vi "LNLS Control PS Data to LOCON_BIPOLAR_16BITS Data_Command9.vi"(8 "error in (no error)":errorcluster, 9 "PS Status (On correction?)":bool[](array[boolean]), 10 "PS Status (ON/OFF)":bool[](array[boolean]), 11 "PS Readings/Setpoints":dbl[](array[numeric])) -> (0 "error out":errorcluster, 3 "PS Readings/Setpoints LOCON Data":T1[](array[typedef]) {"status" format="%08b"})   [LabVIEW 2011, in "LNLS Control VIs.lvlib"]
uses:
  Types Definitions/Type LOCON_BIPOLAR_16BITS.ctl
  LNLS Control VIs.lvlib
  Type Definitions.lvlib
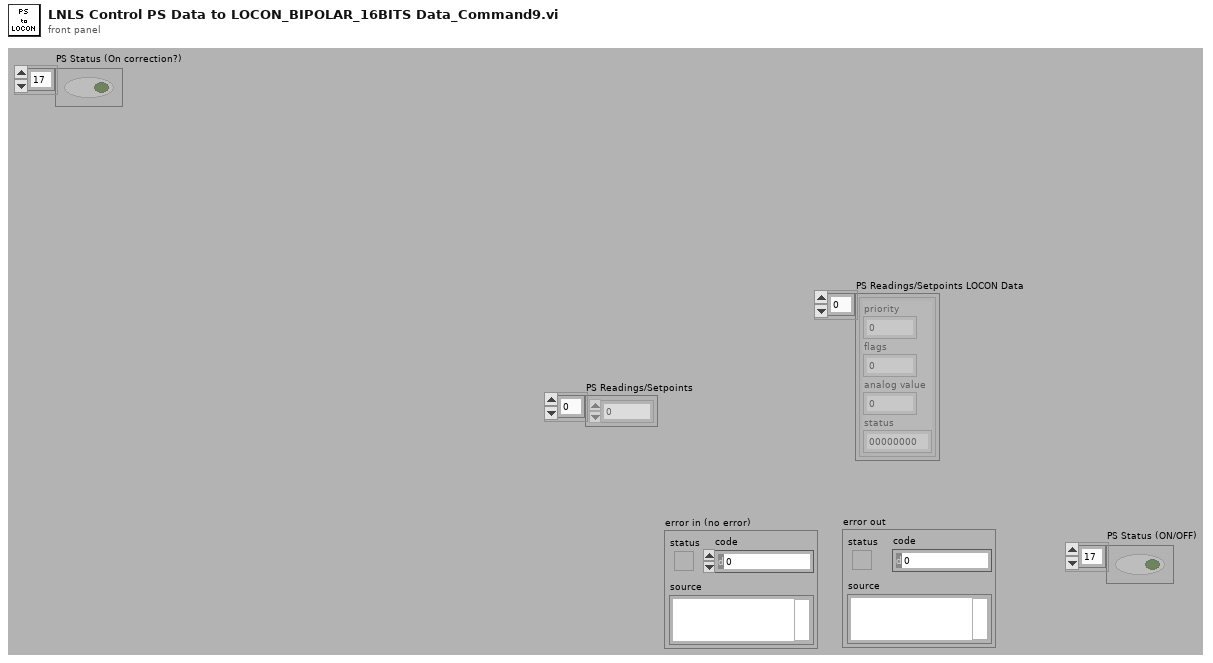
[diagram p1: front panel]
types:
  T1 = typedef "Type Definitions.lvlib/Type LOCON_BIPOLAR_16BITS.ctl" = cluster{"priority":u8, "flags":u8, "analog value":u16, "status":u8}
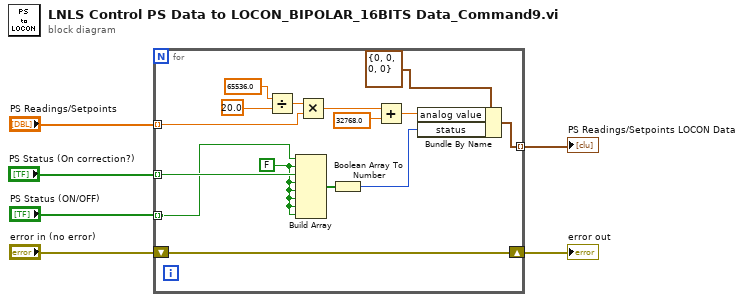
[diagram p0: block diagram]
diagram:
  n1 = for {
    tunnel: [w21] -> w3 mode=indexing
    shift-right: [w15] -> w5
    shift-left: "error in (no error)" -> [w15]
    tunnel: "PS Readings/Setpoints" -> [w12] mode=indexing
    tunnel: "PS Status (ON/OFF)" -> [w8] mode=indexing
    tunnel: "PS Status (On correction?)" -> [w9] mode=indexing
    w7 = FALSE ("element")
    n2 = Divide(x=65536.0, y=20.0) -> (x/y=w14:dbl)
    n3 = Build Array(w8, w7, w9, w7, w7, w7, w7, w7) -> (w11:bool[])
    n4 = Multiply(x=w14, y=w12) -> (x*y=w18:dbl)
    n5 = Boolean Array To Number(Boolean array=w11) -> (number=w10:u32)
    n6 = Add(x=w18, y=32768.0) -> (x+y=w16:dbl)
    n7 = Bundle By Name(cluster=T1 {"priority"=0, "flags"=0, "analog value"=0, "status"=0}, "analog value"=w16, "status"=w10) -> (w21:T1)
  }
  "PS Readings/Setpoints LOCON Data" <- w3
  "error out" <- w5
